vi "Pre Launch Init.vi"(11 "GUI_About in":refnum<class "CalibrationManagerActor.lvclass">) -> (0 "error out":errorcluster, 3 "GUI_About out":refnum<class "CalibrationManagerActor.lvclass">)   [LabVIEW 2017, in "CalibrationManagerActor.lvlib" / "CalibrationManagerActor.lvclass"]
doc: "(<B>Filename</B>: Actor Framework.lvlib:Actor.lvclass:Pre Launch Init.vi)\n\nDefines behavior that occurs after the Launch Nested Actor method is invoked but before the actor's Actor Core method begins running.\n\nBy default, this method does nothing. A descendant class may override it to define behavior."
uses:
  CalibrationManagerActor.lvclass
  CalibrationManagerActor.lvclass/CalibrationManagerActor.ctl
  GUI/GUI/GUI.lvclass
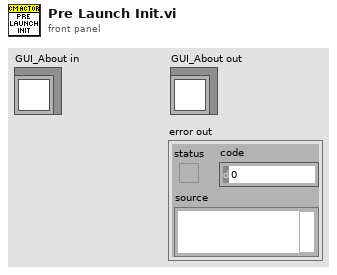
[diagram p1: front panel]
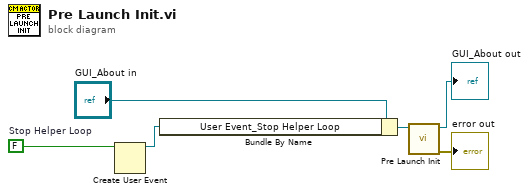
[diagram p0: block diagram]
diagram:
  w3 = FALSE  # Stop Helper Loop
  n1 = Create User Event(user event datatype=w3) -> (user event=w1:refnum<user-event>)  [unwired: 1 in, 1 out]
  n2 = Bundle By Name(cluster="GUI_About in", "User Event_Stop Helper Loop"=w1) -> (w2:refnum<class "CalibrationManagerActor.lvclass">)
  n3 = call-parent "Pre Launch Init.vi"("GUI in"=w2) -> ("error out"=→"error out":errorcluster, "GUI out"=→"GUI_About out":refnum<class "CalibrationManagerActor.lvclass">)  [unwired: 9 in]
